vi "NetImpairFromIni.vi"(8 "ErrorArray In":errorcluster[](array[cluster]), 10 "PathToIni":path, 11 "Bus in":refnum<class "Bus.lvclass">) -> (0 "ErrorArray Out":errorcluster[](array[cluster]), 3 "Bus out":refnum<class "Bus.lvclass">)   [LabVIEW 2017, in "Bus_class.lvlib" / "Bus.lvclass"]
uses:
  Bus.lvclass
  Init/TypeDefs/clInitParams.ctl
  Public/TypeDefs/clBusData.ctl
  FrontPanel/TypeDefs/clEventConfig.ctl
  Modules/PmuImpairPlugins/PmuImpairPluginBase_class/TypeDefs/clImpairConfig.ctl
  Modules/EventPlugins/EventPluginBaseClass/TypeDefs/clEvtReportArray.ctl
  Modules/EventPlugins/EventPluginBaseClass/TypeDefs/clEvtReport.ctl
  Modules/EventPlugins/EventPluginBaseClass/TypeDefs/dblEvtSignalArray.ctl
  Modules/NetworkImpairmentModule/PublicAPI/Arguments/Broadcasts/dblNetworkTime.ctl
  Modules/NetworkImpairmentModule/PublicAPI/Arguments/Broadcasts/dblPktLoss.ctl
  Modules/FlagImpairModule/PublicAPI/Arguments/Broadcasts/ui32FlagImpairmentArray.ctl
  Modules/OutputToFilePlugins/OutputToFileBasePlugin/Typedefs/PmuCfgOpt.ctl
  <vilib>/Utility/config.llb/NI_LVConfig.lvlib
  Framework.lvlib
  Modules/PmuImpairPlugins/PmuImpairPluginBase_class/PmuImpairPluginBase.lvclass
  Modules/EventPlugins/EventPluginBaseClass/EventPluginBaseClass.lvclass
  Modules/NetworkImpairmentModule/NetworkImpairmentModule.lvlib
  Modules/FlagImpairModule/FlagImpairModule.lvlib
  Modules/OutputToFilePlugins/OutputToFileBasePlugin/OutputToFileBasePlugin.lvclass
  <userlib>/NIST/NISTErrorLib/NISTErrorLib.lvlib
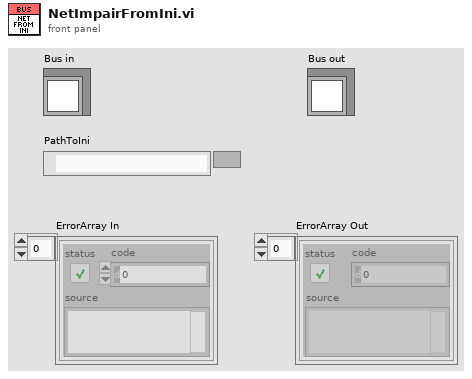
[diagram p1: front panel]
types:
  T1 = typedef "Bus_class.lvlib/Bus.lvclass/clBusData.ctl" = cluster{"BusNumber":u8, "EvtPluginINIFilePath":path, "EvtParams":string[][], "EvtConfig":T2, "Start Time":dbl, "End Time":dbl, "PmuImpairPluginINIFilePath":path, "PmuImpairParams ":string[][], "PmuImpairConfig":T3, "NetImpPluginINIFilePath":path, "NetImpParams":string[][], "FlagImpPluginINIFilePath":path, "FlagImpParams":string[][], "EvtReportArray":T4, "EventSignalArray":T6, "ImpairReportArray":T4, "NetworkTime":T7, "PktLoss":T8, "FlagImpArray":T9, "OutputToFilePluginINIFilePath":path, "Output File Path":path, "clConfigOptions":T10, "AppPluginINIFilePath":path, "AppConfig":variant, "AppOutput":variant}
  T2 = typedef "Framework.lvlib/clEventConfig.ctl" = cluster{"UTC Time 0":timestamp, "Nominal Frequency":u16, "Reporting Rate":u16, "Fsamp":u32, "PosSeq":bool}
  T3 = typedef "PmuImpairPlugins.lvlib/PmuImpairPluginBase.lvclass/clImpairConfig.ctl" = cluster{"FilterType":string, "bPosSeq":bool}
  T4 = typedef "EventPlugins.lvlib/EventPluginBaseClass.lvclass/clEvtReportArray.ctl" = T5[]
  T5 = typedef "EventPlugins.lvlib/EventPluginBaseClass.lvclass/clEvtReport.ctl" = cluster{"Timestamp":dbl, "Synx":cdb[], "Freq":dbl, "ROCOF":dbl, "ID":i16}
  T6 = typedef "EventPlugins.lvlib/EventPluginBaseClass.lvclass/dblEvtSignalArray.ctl" = dbl[][]
  T7 = typedef "NetworkImpairmentModule.lvlib/dblNetworkTime.ctl" = dbl[]
  T8 = typedef "NetworkImpairmentModule.lvlib/dblPktLoss.ctl" = dbl[]
  T9 = typedef "FlagImpairModule.lvlib/ui32FlagImpairmentArray.ctl" = u32[]
  T10 = typedef "OutputToFilePlugins.lvlib/OutputToFileBasePlugin.lvclass/PmuCfgOpt.ctl" = cluster{"TIME_BASE":u64, "STN":string, "IDCODE":u16, "rdoPolRect":enum32{"Rectangular", "Polar"}, "rdoFloatInt":enum32{"Float", "Integer"}, "PHUNIT":u64, "rdoFreqDfreq":enum32{"Float", "Integer"}, "CHNAM":string[], "chkCfg2Prefix":bool}
  T11 = typedef "Framework.lvlib/clInitParams.ctl" = cluster{"RowHdrs":string[], "ColHdrs":string[], "DefaultParams":string[][]}
  T12 = typedef "NI_LVConfig.lvlib/Config Data RefNum.ctl" = refnum<k1>
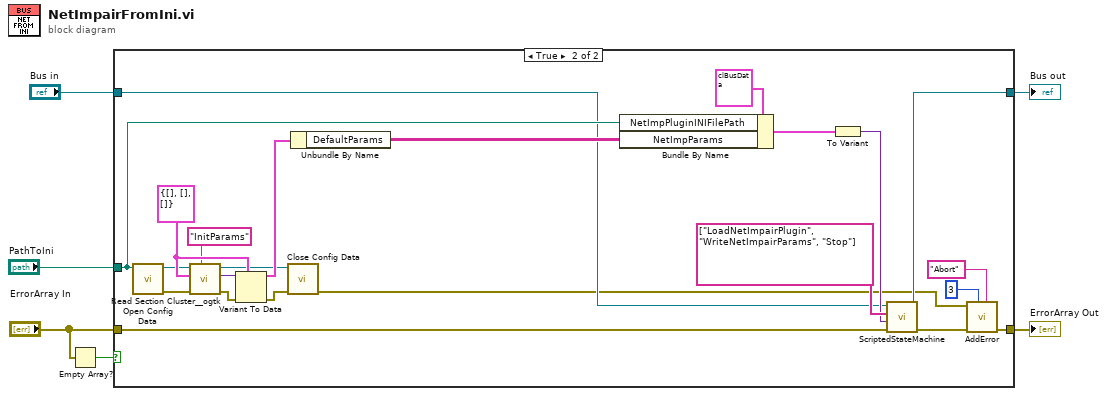
[diagram p0: block diagram]
diagram:
  n1 = Empty Array?(array="ErrorArray In") -> (empty?=w5:bool)
  n2 = case shown="True" w5 {
    tunnel: "ErrorArray In" -> [w8 w11]
    tunnel: [w8 w17] -> w4
    tunnel: "Bus in" -> [w7 w12]
    tunnel: [w7 w19] -> w2
    tunnel: "PathToIni" -> [_ w23]
    frame False {
    }
    frame True {
      w31 = T11 {"RowHdrs"=[], "ColHdrs"=[], "DefaultParams"=[]} ("ParamsHdrs")
      n3 = call <vilib>:"Open Config Data.vi"("configuration file path"=w23) -> ("error out"=w26:errorcluster, "refnum"=w27:T12)  [unwired: 8 in, 1 out]
      n4 = call <userlib>:"Read Section Cluster__ogtk.vi"("section (optional)"="InitParams", "error in (no error)"=w26, "Section Formatted Cluster Type"=w31, "refnum"=w27) -> ("error out"=w29:errorcluster, "Section Formatted Cluster"=w30:variant, "dup refnum"=w13:T12)  [unwired: 3 in, 2 out]
      n5 = Variant To Data(error in=w29, type=w31, Variant=w30) -> (data=w25:T11, error out=w14:errorcluster)
      n6 = call <vilib>:"Close Config Data.vi"("error in (no error)"=w14, "refnum"=w13) -> ("error out"=w9:errorcluster)  [unwired: 8 in, 1 out]
      n7 = Unbundle By Name(w25) -> ("DefaultParams"=w24:string[][])
      n8 = Bundle By Name(cluster=T1 {"BusNumber"=0, "EvtPluginINIFilePath"=path "", "EvtParams"=[], "EvtConfig"={"UTC Time 0"=timestamp(0 s since 1904-01-01), "Nominal Frequency"=60, "Reporting Rate"=60, "Fsamp"=960, "PosSeq"=FALSE}, "Start Time"=0.0, "End Time"=0.0, "PmuImpairPluginINIFilePath"=path "", "PmuImpairParams "=[["960"], ["8.19"], ["164"]], "PmuImpairConfig"={"FilterType"="", "bPosSeq"=TRUE}, "NetImpPluginINIFilePath"=path "", "NetImpParams"=[], "FlagImpPluginINIFilePath"=path "", "FlagImpParams"=[], "EvtReportArray"=[], "EventSignalArray"=[], "ImpairReportArray"=[], "NetworkTime"=[], "PktLoss"=[], "FlagImpArray"=[], "OutputToFilePluginINIFilePath"=path "", "Output File Path"=path "", "clConfigOptions"={"TIME_BASE"=1000000, "STN"="Bus_1", "IDCODE"=0, "rdoPolRect"=enum."Rectangular", "rdoFloatInt"=enum."Float", "PHUNIT"=1000000, "rdoFreqDfreq"=enum."Float", "CHNAM"=["VA", "VB", "VC", "V+", "IA", "IB", "IC", "I+"], "chkCfg2Prefix"=TRUE}, "AppPluginINIFilePath"=path "", "AppConfig"=variant, "AppOutput"=variant} ("clBusData"), "NetImpPluginINIFilePath"=w23, "NetImpParams"=w24) -> (w21:T1)
      n9 = To Variant(anything=w21) -> (Variant=w20:variant)
      n10 = call "ScriptedStateMachine.vi"("ErrorArray In"=w11, "Data in"=w20, "Script"=string[] ["LoadNetImpairPlugin", "WriteNetImpairParams", "Stop"], "Bus"=w12) -> ("ErrorArray Out"=w18:errorcluster[], "Bus"=w19:refnum<class "Bus.lvclass">)  [unwired: 5 in, 1 out]
      n11 = call <userlib>:"AddError.vi"("Severity"="Abort", "Priority"=u8 3, "ErrorArray"=w18, "error in (no error)"=w9) -> ("ErrorArray"=w17:errorcluster[])  [unwired: 6 in, 1 out]
    }
  }
  "ErrorArray Out" <- w4
  "Bus out" <- w2
